vi "SpreadSheetStringToArray_CleanEmptyFieldsAtTheEnd.vi"(7 "SpreadSheetString.In":string) -> (6 "SpreadSheetString.OUT":string, 10 "SpreadSheetArray.OUT":string[](array[string]))   [LabVIEW 2024]
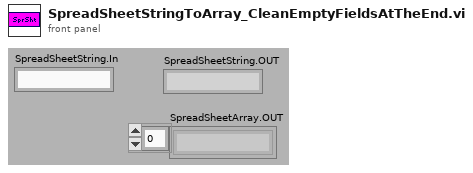
[diagram p1: front panel]
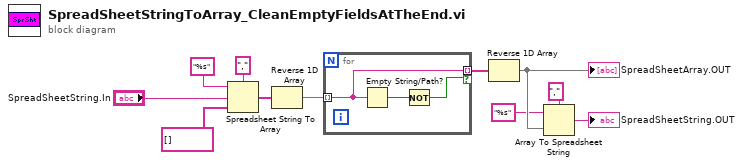
[diagram p0: block diagram]
diagram:
  n1 = Spreadsheet String To Array(delimiter (Tab)=",", format string="%s" ("spreadsheet string"), spreadsheet string="SpreadSheetString.In", array type (2D Dbl)=string[] []) -> (array=w7:string[])
  n2 = Reverse 1D Array(array=w7) -> (reversed array=w6:string[])
  n3 = for {
    tunnel: w6 -> [w14] mode=indexing
    tunnel: [w14] -> w1 mode=indexing if=w12
    n4 = Empty String/Path?(string/path=w14) -> (empty?=w13:bool)
    n5 = Not(x=w13) -> (.not. x?=w12:bool)
  }
  n6 = Reverse 1D Array(array=w1) -> (reversed array=w5:string[])
  "SpreadSheetArray.OUT" <- w5
  n7 = Array To Spreadsheet String(delimiter (Tab)=",", array=w5, 3:"%s" ("format string")) -> (spreadsheet string=→"SpreadSheetString.OUT":string)
